vi "automatic_step_address.vi"(7 "transition_queue":refnum<queue>, 8 "error in (no error)":errorcluster, 10 "data":variant, 11 "recipe_data":variant) -> (0 "error out":errorcluster)   [LabVIEW 2015, in "example_02.lvlib"]
uses:
  example_02.lvlib
  <userlib>/antonio-alexander/lv-recipe-machine/public/_controls/transition.ctl
  _controls/customer.ctl
  <userlib>/antonio-alexander/lv-recipe-machine/lv-recipe-machine.lvlib
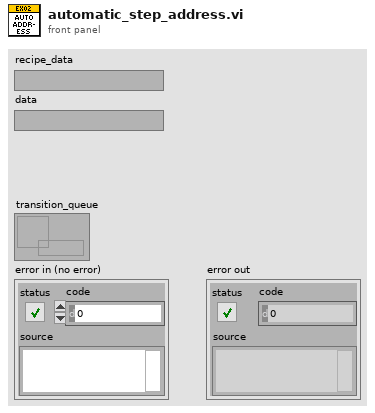
[diagram p1: front panel]
types:
  T1 = typedef "example_02.lvlib/customer.ctl" = cluster{"first_name":string, "last_name":string, "address_1":string, "address_2":string, "city":string, "state":string, "zip_code":string}
  T2 = typedef "example_02.lvlib/data.ctl" = cluster{"type":T3, "data":variant}
  T3 = typedef "example_02.lvlib/data_type.ctl" = enum16{"<data_type>", "first_name", "last_name", "address", "city", "state", "zip_code"}
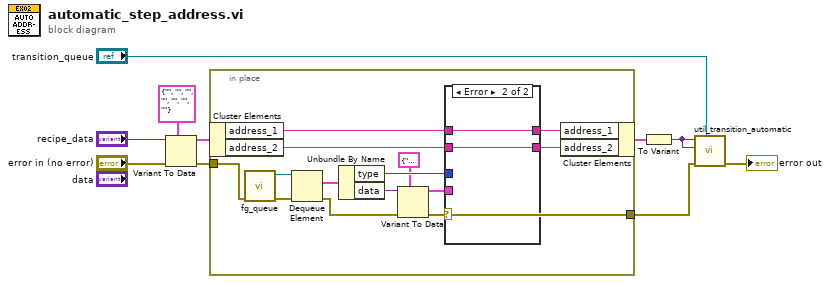
[diagram p0: block diagram]
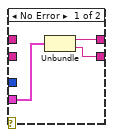
[diagram p2: hidden frame]
diagram:
  n1 = Variant To Data(error in="error in (no error)", type=T1 {"first_name"="", "last_name"="", "address_1"="", "address_2"="", "city"="", "state"="", "zip_code"=""} ("customer"), Variant="recipe_data") -> (data=w5:T1, error out=w2:errorcluster)
  n2 = in-place {
    in-place-border: w2 -> [w22]
    in-place-border: [w17] -> w1
    n3 = in-place-cluster #1(w5) -> ("address_1"=w18:string, "address_2"=w13:string)
    n4 = call "fg_queue.vi"("error in (no error)"=w22) -> ("error out"=w23:errorcluster, "queue out"=w24:refnum<queue>)  [unwired: 9 in]
    n5 = Dequeue Element(queue=w24, error in (no error)=w23) -> (element=w21:T2, error out=w19:errorcluster)  [unwired: 1 in, 2 out]
    n6 = Unbundle By Name(w21) -> ("type"=w14:T3, "data"=w20:variant)
    n7 = Variant To Data(error in=w19, type=cluster{string, string} {"", ""}, Variant=w20) -> (data=w16:cluster{string, string}, error out=w17:errorcluster)
    n8 = case shown="Error" w17 {
      tunnel: w18 -> [_ w29]
      tunnel: w16 -> [w27 _]
      tunnel: [w26 w29] -> w15
      tunnel: w14 -> [_ _]
      tunnel: w13 -> [_ w28]
      tunnel: [w25 w28] -> w11
      frame No Error {
        n9 = Unbundle(w27) -> (w26:string, w25:string)
      }
      frame Error {
      }
    }
    n10 = in-place-cluster #1("address_1"=w15, "address_2"=w11) -> (w4:T1)
  }
  n11 = To Variant(anything=w4) -> (Variant=w3:variant)
  n12 = call <userlib>:"util_transition_automatic.vi"("transition_queue"="transition_queue", "error in (no error)"=w1, "data"=w3, "recipe_data"=w3) -> ("error out"=→"error out":errorcluster)  [unwired: 7 in]
